vi "Read_Table_Result.vi"(0 "Condition Test":string(combo)="D_L", 3 "Number Product":i32) -> (5 "Row Number":i32, 6 "File name.":path, 7 "Path Ready":bool, 8 "all rows":string[][](array[string]), 9 "String Result":string, 10 "Num Result":u8)   [LabVIEW 2017]
uses:
  <vilib>/Utility/file.llb/Read Delimited Spreadsheet (string).vi
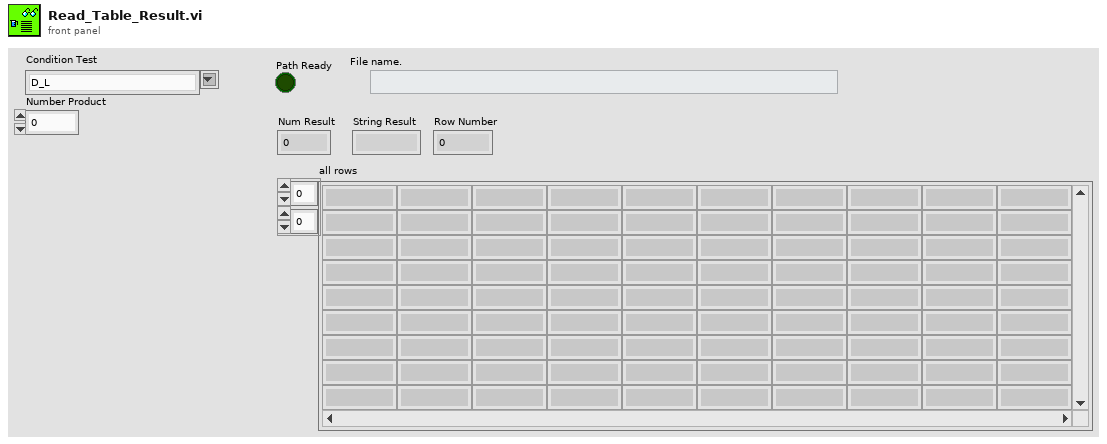
[diagram p1: front panel]
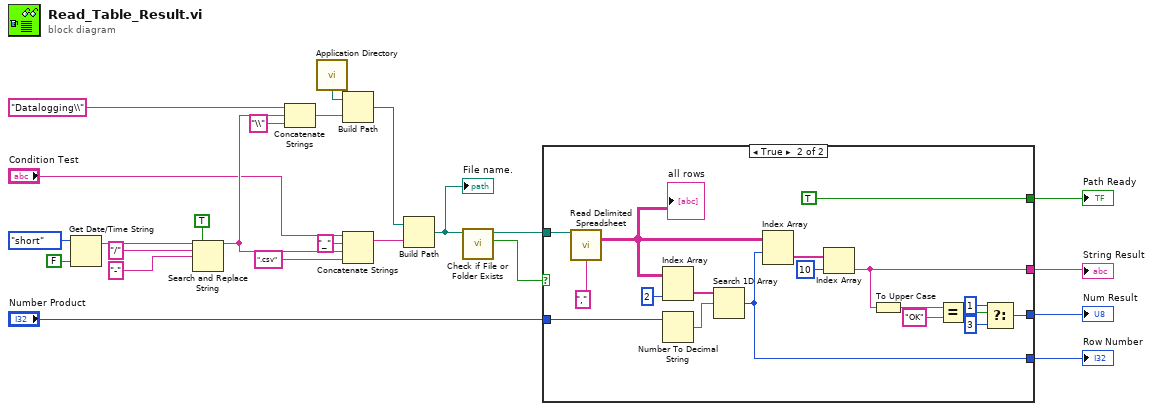
[diagram p0: block diagram]
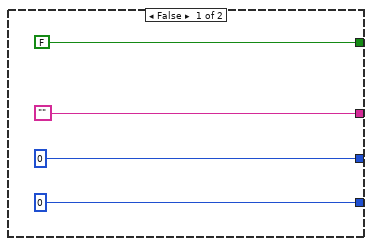
[diagram p2: hidden frame]
diagram:
  n1 = Get Date/Time String(date format (0)=enum16{"short", "long", "abbreviated"}."short", want seconds? (F)=FALSE) -> (date string=w4:string)  [unwired: 1 in, 1 out]
  n2 = Search and Replace String(replace all?=TRUE ("replace all? (F)"), input string=w4, search string="/" ("input string"), replace string="-" ("replace string (\"\")")) -> (result string=w11:string)  [unwired: 4 in, 3 out]
  n3 = Concatenate Strings("Datalogging\\", w11, "\\" ("string")) -> (w8:string)
  n4 = call <vilib>:"Application Directory.vi"() -> ("Application Directory"=w9:path)
  n5 = Build Path(base path=w9, name or relative path=w8) -> (appended path=w7:path)
  n6 = Concatenate Strings("Condition Test", "_" ("string"), w11, ".csv" ("string")) -> (w13:string)
  n7 = Build Path(base path=w7, name or relative path=w13) -> (appended path=w3:path)
  "File name." <- w3
  n8 = call <vilib>:"Check if File or Folder Exists.vi"("path"=w3) -> ("file or folder exists?"=w19:bool, "dup path"=w20:path)  [unwired: 8 in, 1 out]
  n9 = case shown="True" w19 {
    tunnel: w20 -> [_ w40]
    tunnel: "Number Product" -> [_ w35]
    tunnel: ["" w44] -> w21
    tunnel: [FALSE TRUE] -> w18
    tunnel: [0 ("index of element") w33] -> w2
    tunnel: [u8 0 ("f") w29] -> w1
    frame False {
    }
    frame True {
      n10 = call-poly <vilib>:"Read Delimited Spreadsheet.vi"("file path (dialog if empty)"=w40, "delimiter (\\t)"="," ("delimiter (\\t)")) -> ("all rows"=w38:string[][])  [unwired: 8 in, 5 out]
      "all rows" <- w38
      n11 = Index Array(array=w38, index (col)=2 ("disabled index (col)")) -> (element=w36:string[])  [unwired: 1 in]
      n12 = Number To Decimal String(number=w35) -> (decimal integer string=w34:string)  [unwired: 1 in]
      n13 = Search 1D Array(1D array=w36, element=w34) -> (index of element=w33:i32)  [unwired: 1 in]
      n14 = Index Array(array=w38, index (row)=w33) -> (element=w46:string[])  [unwired: 1 in]
      n15 = Index Array(array=w46, index=10) -> (element=w44:string)
      n16 = To Upper Case(1:w44) -> (0:w43:string)
      n17 = Equal?(x=w43, y="OK") -> (x = y?=w32:bool)
      n18 = Select(t=u8 1, s=w32, f=u8 3) -> (s? t:f=w29:u8)
    }
  }
  "String Result" <- w21
  "Path Ready" <- w18
  "Row Number" <- w2
  "Num Result" <- w1
